vi "TypeCharacters.vi"(2 "error in (no error) 2":errorcluster, 3 "Length of Key Press (ms)":u32, 4 "Key Array":T1(array[cluster])) -> (0 "error out":errorcluster)   [LabVIEW 2013]
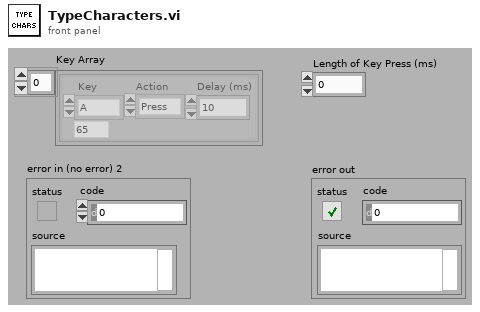
[diagram p1: front panel]
types:
  T1 = cluster{" Key":u8, "Action":enum16{"Press", "Up", "Down"}, "Delay (ms)":u32}[]
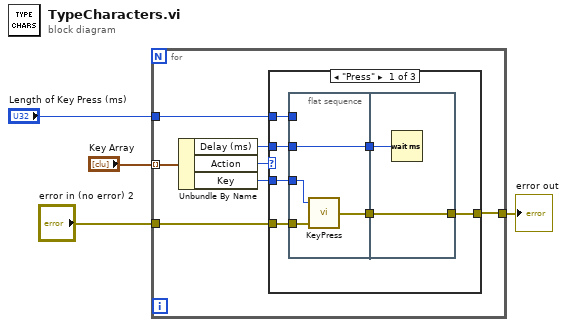
[diagram p0: block diagram]
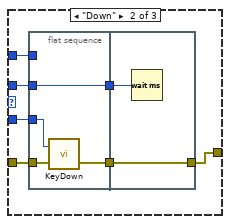
[diagram p2: hidden frame]
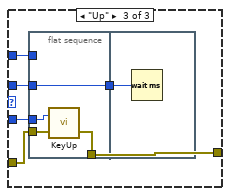
[diagram p3: hidden frame]
diagram:
  n1 = for {
    tunnel: "Key Array" -> [w11] mode=indexing
    tunnel: "Length of Key Press (ms)" -> [w10]
    tunnel: [w6] -> w1
    tunnel: "error in (no error) 2" -> [w5]
    n2 = Unbundle By Name(w11) -> ("Delay (ms)"=w7:u32, "Action"=w9:enum16{"Press", "Up", "Down"}, "Key"=w8:u8)
    n3 = case shown="\"Press\"" w9 {
      tunnel: w10 -> [w18 w31 w43]
      tunnel: w8 -> [w17 w30 w42]
      tunnel: w7 -> [w15 w28 w40]
      tunnel: [w13 w25 w38] -> w6
      tunnel: w5 -> [w14 w27 w39]
      frame "Press" {
        n4 = flat-sequence {
          tunnel: w18 -> [_]
          tunnel: w17 -> [w22]
          tunnel: [w21] -> w16
          tunnel: w15 -> [w21]
          tunnel: w14 -> [w20]
          tunnel: [w19] -> w12
          tunnel: w16 -> [w24]
          tunnel: [w23] -> w13
          tunnel: w12 -> [w23]
          frame #0 {
            n5 = call "KeyPress.vi"("error in (no error)"=w20, "Virtual Key"=w22) -> ("error out"=w19:errorcluster)  [unwired: 1 in]
          }
          frame #1 {
            n6 = Wait (ms)(milliseconds to wait=w24) -> ()  [unwired: 1 out]
          }
        }
      }
      frame "Down" {
        n7 = flat-sequence {
          tunnel: w31 -> [_]
          tunnel: w30 -> [w35]
          tunnel: [w34] -> w29
          tunnel: w28 -> [w34]
          tunnel: w27 -> [w33]
          tunnel: [w32] -> w26
          tunnel: w29 -> [w37]
          tunnel: w26 -> [w36]
          tunnel: [w36] -> w25
          frame #0 {
            n8 = call "KeyDown.vi"("error in (no error)"=w33, "Virtual Key"=w35) -> ("error out"=w32:errorcluster)  [unwired: 1 in]
          }
          frame #1 {
            n9 = Wait (ms)(milliseconds to wait=w37) -> ()  [unwired: 1 out]
          }
        }
      }
      frame "Up" {
        n10 = flat-sequence {
          tunnel: w43 -> [_]
          tunnel: w42 -> [w47]
          tunnel: [w46] -> w41
          tunnel: w40 -> [w46]
          tunnel: w39 -> [w45]
          tunnel: [w44] -> w38
          tunnel: w41 -> [w48]
          frame #0 {
            n11 = call "KeyUp.vi"("error in (no error)"=w45, "Virtual Key"=w47) -> ("error out"=w44:errorcluster)  [unwired: 1 in]
          }
          frame #1 {
            n12 = Wait (ms)(milliseconds to wait=w48) -> ()  [unwired: 1 out]
          }
        }
      }
    }
  }
  "error out" <- w1
